vi "Actor Core.vi"(8 "error in":errorcluster, 11 "Hardware in":refnum<class "mcl_panel.lvclass">) -> (0 "error out":errorcluster, 3 "Actor out":refnum<class "Actor.lvclass">)   [LabVIEW 2015, in "mcl_panel.lvclass"]
doc: "(<B>Filename</B>: Actor Framework.lvlib:Actor.lvclass:Actor Core.vi)\n\nReceives messages to the actor, reacts to them, and initiates any error handling that may shut the actor down.\n\nDescendant classes may override this VI to append parallel tasks for the actor to complete while it handles messages. Overrides use the Call Parent Method node."
uses:
  mcl_panel.lvclass
  <vilib>/ActorFramework/Actor/Actor.lvclass
  UI/panel_class/panel.lvclass/panel.ctl
  <vilib>/ActorFramework/Actor/Actor.lvclass/Actor.ctl
  <vilib>/ActorFramework/Message Enqueuer/Message Enqueuer.lvclass/Message Enqueuer.ctl
  mcl_panel Messages/mcl_move_piezos Msg/mcl_move_piezos Msg.lvclass/mcl_move_piezos Msg.ctl
  <vilib>/ActorFramework/Message Enqueuer/Init from Existing Queue.vi
  <vilib>/ActorFramework/Message Enqueuer/Enqueue.vi
  <vilib>/ActorFramework/Message Priority Queue/Priority Enqueue.vi
  <vilib>/ActorFramework/Message Enqueuer/Message Enqueuer.lvclass
  mcl_panel Messages/mcl_move_piezos Msg/mcl_move_piezos Msg.lvclass
  mcl_panel Messages/mcl_connect Msg/mcl_connect Msg.lvclass
  mcl_panel Messages/mcl_query_positions Msg/mcl_query_positions Msg.lvclass
  UI/panel_class/panel.lvclass
panel:
  in  "Scratch":string
  in  "copy_coors":bool
  in  "step":dbl
  in  "right":bool
  in  "left":bool
  in  "down":bool
  in  "up":bool
  out "Z":dbl
  out "Y":dbl
  out "X":dbl
  in  "Speed":dbl
  in  "move_kinesis":bool
  in  "Z":dbl
  in  "Y":dbl
  in  "X":dbl
  out "Status":string
  in  "connect_mcl":bool
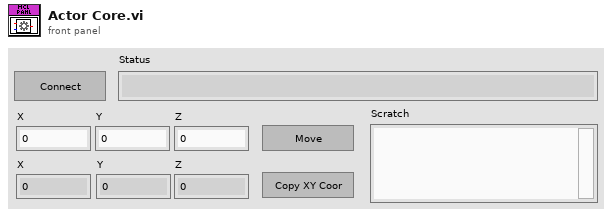
[diagram p1: front panel]
types:
  T1 = typedef "thorlabs_event_refs.ctl" = cluster{"Event Registration Refnum":refnum<event-registration>, "Event Registration Refnum":refnum<event-registration>}
  T2 = cluster{"Event Registration Refnum":refnum<event-registration>, "stop_ui_ref":refnum<event-registration>, "Event Registration Refnum":refnum<event-registration>}
  T3 = typedef "ui_plot_references.ctl" = cluster{"plots":refnum<vi>, "chart":refnum<vi>, "graph":refnum<vi>, "map":refnum<vi>, "XY Graph":refnum<vi>}
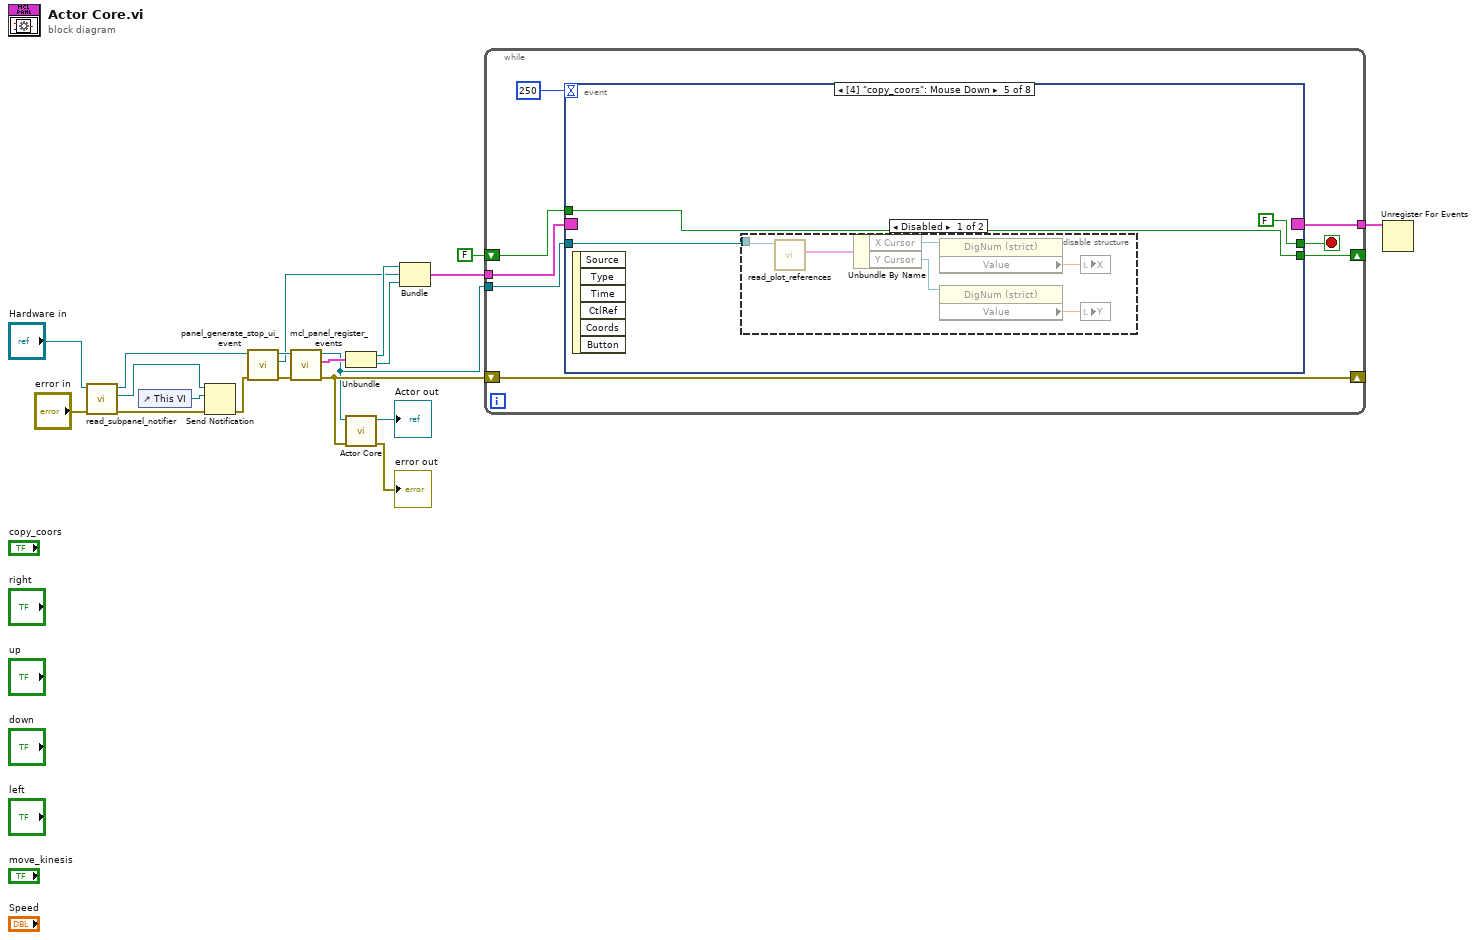
[diagram p0: block diagram]
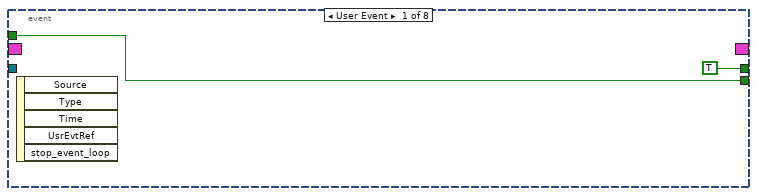
[diagram p2: hidden frame]
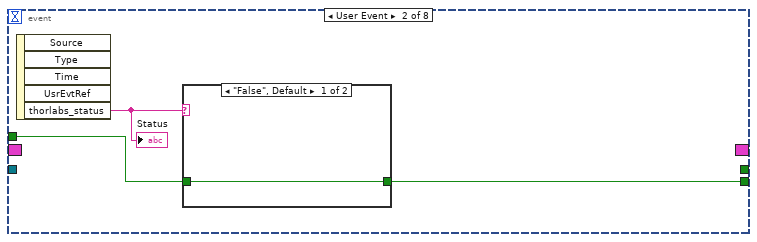
[diagram p3: hidden frame]
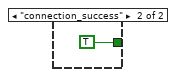
[diagram p4: hidden frame]
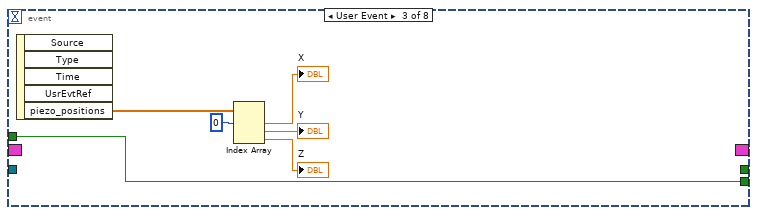
[diagram p5: hidden frame]
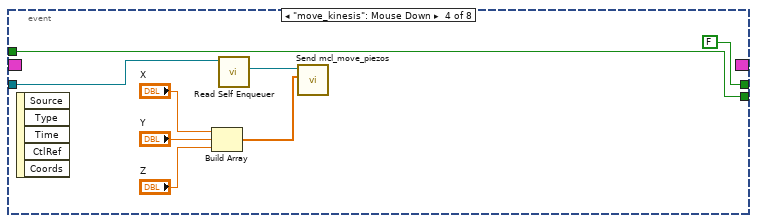
[diagram p6: hidden frame]
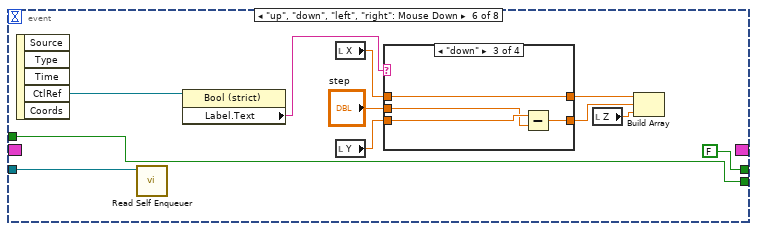
[diagram p8: hidden frame]
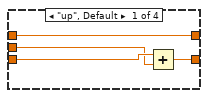
[diagram p9: hidden frame]
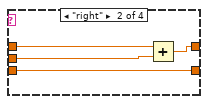
[diagram p10: hidden frame]
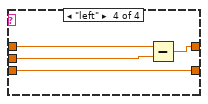
[diagram p11: hidden frame]
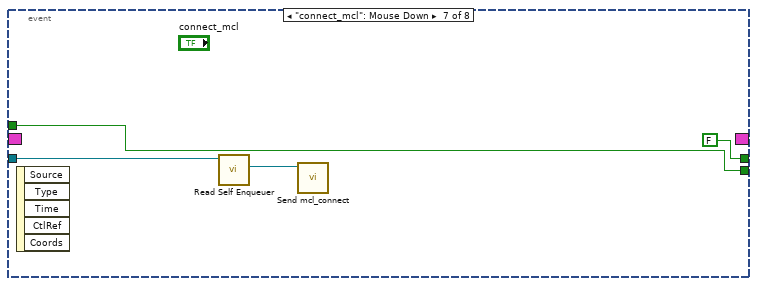
[diagram p12: hidden frame]
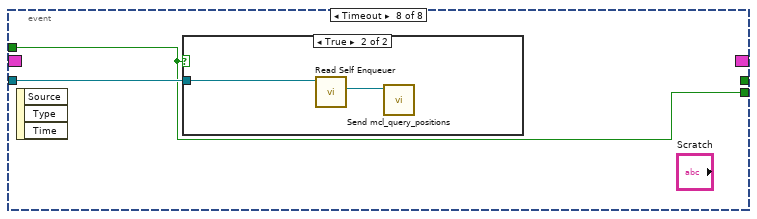
[diagram p13: hidden frame]
diagram:
  n1 = call "read_subpanel_notifier.vi"("error in (no error)"="error in", "panel in"="Hardware in") -> ("error out"=w14:errorcluster, "subpanel_notifier"=w16:refnum<notifier>, "panel out"=w15:refnum<class "mcl_panel.lvclass">)  [unwired: 7 in]
  n2 = control-ref of="This VI"() -> (w18:refnum<vi>)
  n3 = Send Notification(notification=w18, notifier=w16, error in (no error)=w14) -> (error out=w13:errorcluster)  [unwired: 1 out]
  n4 = call "panel_generate_stop_ui_event.vi"("error in (no error)"=w13, "panel in"=w15) -> ("error out"=w9:errorcluster, "stop_ui_ref"=w5:refnum<event-registration>, "panel out"=w10:refnum<class "mcl_panel.lvclass">)  [unwired: 7 in]
  n5 = call "mcl_panel_register_events.vi"("error in (no error)"=w9, "thorlabs_panel in"=w10) -> ("error out"=w8:errorcluster, "event_refs cluster"=w7:T1, "thorlabs_panel out"=w2:refnum<class "mcl_panel.lvclass">)  [unwired: 7 in]
  n6 = Unbundle(w7) -> ("Event Registration Refnum"=w6:refnum<event-registration>, "Event Registration Refnum"=w4:refnum<event-registration>)
  n7 = call-parent "Actor Core.vi"("error in"=w8, "Actor in"=w2) -> ("error out"=→"error out":errorcluster, "Actor out"=→"Actor out":refnum<class "Actor.lvclass">)  [unwired: 8 in]
  n8 = Bundle("Event Registration Refnum"=w6, "stop_ui_ref"=w5, "Event Registration Refnum"=w4) -> (w3:T2)  [unwired: 1 in]
  n9 = while {
    tunnel: w3 -> [w28]
    tunnel: [w26] -> w11
    shift-right: [w25] -> _
    shift-left: w8 -> [w25]
    tunnel: w2 -> [w24]
    shift-right: [w21] -> _
    shift-left: FALSE -> [w22]
    stop <- w27 stop-if-true
    n10 = event shown="[4] \"copy_coors\": Mouse Down" {
      selector: w28 -> [_ _ _ _ _ _ _ _]
      dyn-events: [_ _ _ _ _ _ _ _] -> w26
      timeout: 250 -> [_ _ _ _ _ _ _ _]
      tunnel: [TRUE _ _ FALSE FALSE FALSE FALSE _] -> w27
      tunnel: w24 -> [_ _ _ w49 w52 w61 w89 w91]
      tunnel: w22 -> [w29 w32 w36 w44 w50 w60 w87 w90]
      tunnel: [w29 w31 w36 w44 w50 w60 w87 w90] -> w21
      event User Event {
        n11 = event-data() -> ()  [unwired: 1 in, 5 out]
      }
      event User Event {
        n12 = event-data() -> ("thorlabs_status"=w33:string)  [unwired: 1 in, 4 out]
        "Status" <- w33
        n13 = case shown="\"False\", Default" w33 {
          tunnel: w32 -> [w34 _]
          tunnel: [w34 TRUE] -> w31
          frame "False", Default {
          }
          frame "connection_success" {
          }
        }
      }
      event User Event {
        n14 = event-data() -> ("piezo_positions"=w41:dbl[])  [unwired: 1 in, 4 out]
        n15 = Index Array(array=w41, index #1=0 ("index")) -> (element #1=→"X":dbl, element #2=→"Y":dbl, element #3=→"Z":dbl)  [unwired: 2 in]
      }
      event "move_kinesis": Mouse Down {
        n16 = event-data() -> ()  [unwired: 1 in, 5 out]
        n17 = Build Array("X", "Y", "Z") -> (w42:dbl[])
        n18 = call <vilib>:"Read Self Enqueuer.vi"("Actor"=w49) -> ("Self Enqueuer"=w43:refnum<class "Message Enqueuer.lvclass">)  [unwired: 10 in]
        n19 = call "Send mcl_move_piezos.vi"("new_positions"=w42, "Message Enqueuer"=w43) -> ()  [unwired: 8 in, 2 out]
      }
      event "copy_coors": Mouse Down {
        n20 = event-data() -> ()  [unwired: 1 in, 6 out]
        n21 = disable-structure shown="Disabled" {
          disable-tunnel: w52 -> [w58 _]
          frame Disabled {
            n22 = call "read_plot_references.vi"("panel in"=w58) -> ("plot_references"=w57:T3)  [unwired: 8 in, 2 out]
            n23 = Unbundle By Name(w57) -> ("X Cursor"=w56:refnum<vi>, "Y Cursor"=w54:refnum<vi>)
            n24 = property class="DigNum (strict)"(reference=w56) -> ("Value"=w55:dbl)  [unwired: 1 in, 2 out]
            n25 = property class="DigNum (strict)"(reference=w54) -> ("Value"=w53:dbl)  [unwired: 1 in, 2 out]
            n26 = local write "X"(w55) -> ()
            n27 = local write "Y"(w53) -> ()
          }
          frame Enabled {
          }
        }
      }
      event "up", "down", "left", "right": Mouse Down {
        n28 = event-data() -> ("CtlRef"=w69:refnum<vi>)  [unwired: 1 in, 4 out]
        n29 = call <vilib>:"Read Self Enqueuer.vi"("Actor"=w61) -> ()  [unwired: 10 in, 1 out]
        n30 = property class="Bool (strict)"(reference=w69) -> ("Label.Text"=w68:string)  [unwired: 1 in, 2 out]
        n31 = local read "X"() -> (w63:dbl)
        n32 = local read "Y"() -> (w66:dbl)
        n33 = case shown="\"down\"" w68 {
          tunnel: w66 -> [w73 w74 w81 w82]
          tunnel: "step" -> [w72 w77 w80 w85]
          tunnel: [w71 w74 w79 w82] -> w64
          tunnel: w63 -> [w70 w76 w78 w84]
          tunnel: [w70 w75 w78 w83] -> w62
          frame "up", Default {
            n34 = Add(x=w73, y=w72) -> (x+y=w71:dbl)
          }
          frame "right" {
            n35 = Add(x=w76, y=w77) -> (x+y=w75:dbl)
          }
          frame "down" {
            n36 = Subtract(x=w81, y=w80) -> (x-y=w79:dbl)
          }
          frame "left" {
            n37 = Subtract(x=w84, y=w85) -> (x-y=w83:dbl)
          }
        }
        n38 = local read "Z"() -> (w67:dbl)
        n39 = Build Array(w62, w64, w67) -> ()  [unwired: 1 out]
      }
      event "connect_mcl": Mouse Down {
        n40 = event-data() -> ()  [unwired: 1 in, 5 out]
        n41 = call <vilib>:"Read Self Enqueuer.vi"("Actor"=w89) -> ("Self Enqueuer"=w86:refnum<class "Message Enqueuer.lvclass">)  [unwired: 10 in]
        n42 = call "Send mcl_connect.vi"("Message Enqueuer"=w86) -> ()  [unwired: 9 in, 2 out]
      }
      event Timeout {
        n43 = event-data() -> ()  [unwired: 1 in, 3 out]
        n44 = case shown="True" w90 {
          tunnel: w91 -> [_ w93]
          frame False {
          }
          frame True {
            n45 = call <vilib>:"Read Self Enqueuer.vi"("Actor"=w93) -> ("Self Enqueuer"=w92:refnum<class "Message Enqueuer.lvclass">)  [unwired: 10 in]
            n46 = call "Send mcl_query_positions.vi"("Message Enqueuer"=w92) -> ()  [unwired: 9 in, 2 out]
          }
        }
      }
    }
  }
  n47 = Unregister For Events(event registration refnum=w11) -> ()  [unwired: 1 in, 1 out]
